vi "Position Cancel Key.vi"(8 "error in (no error)":errorcluster, 10 "Space Bar Key":refnum<vi>, 11 "Done Key":refnum<vi>) -> (0 "error out":errorcluster)   [LabVIEW 2014]
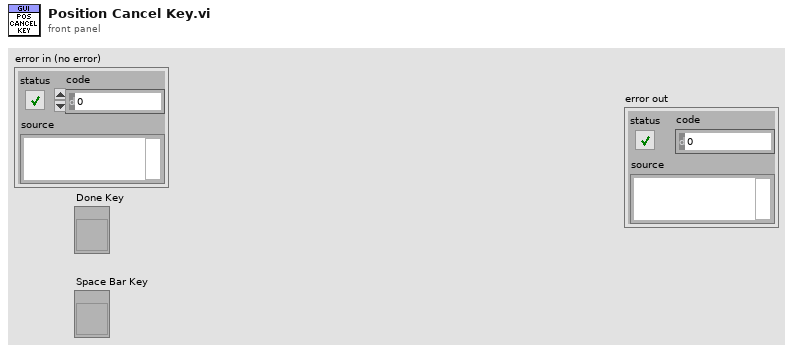
[diagram p1: front panel]
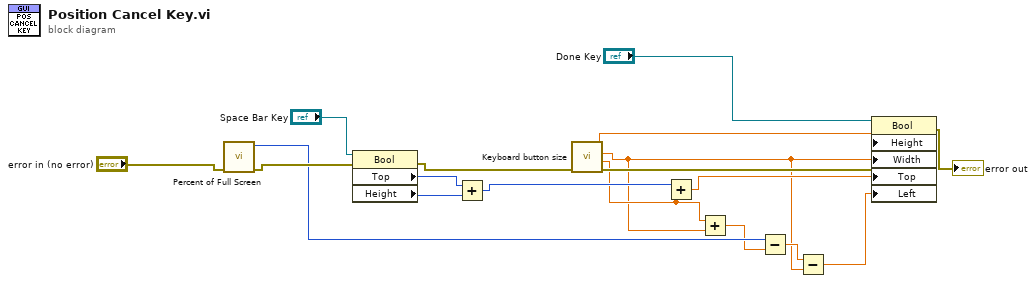
[diagram p0: block diagram]
diagram:
  n1 = call "Percent of Full Screen.vi"("error in (no error)"="error in (no error)") -> ("error out"=w7:errorcluster, "Right"=w5:i16)  [unwired: 8 in, 1 out]
  n2 = property class="Bool"(reference="Space Bar Key", error in=w7) -> (error out=w14:errorcluster, "Top"=w12:i32, "Height"=w11:u32)  [unwired: 1 out]
  n3 = Add(x=w12, y=w11) -> (x+y=w10:u32)
  n4 = call "Keyboard button size.vi"("error in (no error)"=w14) -> ("error out"=w17:errorcluster, "Key Spacing"=w8:dbl, "Key Width"=w2:dbl, "Key Height"=w15:dbl)  [unwired: 7 in]
  n5 = Add(x=w10, y=w8) -> (x+y=w9:dbl)
  n6 = Add(x=w8, y=w2) -> (x+y=w4:dbl)
  n7 = Subtract(x=w5, y=w4) -> (x-y=w3:dbl)
  n8 = Subtract(x=w3, y=w2) -> (x-y=w1:dbl)
  n9 = property class="Bool"(reference="Done Key", error in=w17, "Height"=w15, "Width"=w2, "Top"=w9, "Left"=w1) -> (error out=→"error out":errorcluster)  [unwired: 1 out]
